vi "find_element(array).vi"(8 "error in (no error)":errorcluster, 10 "name":string, 11 "data store (in)":cluster{"name":string, "address":string}[](array[cluster])) -> (0 "error out":errorcluster, 1 "element":cluster{"name":string, "address":string}, 2 "element found ?":bool, 3 "data store (out)":cluster{"name":string, "address":string}[](array[cluster]))   [LabVIEW 2018]
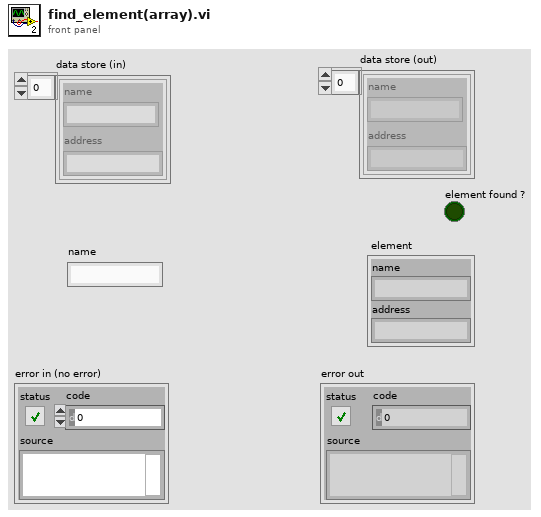
[diagram p1: front panel]
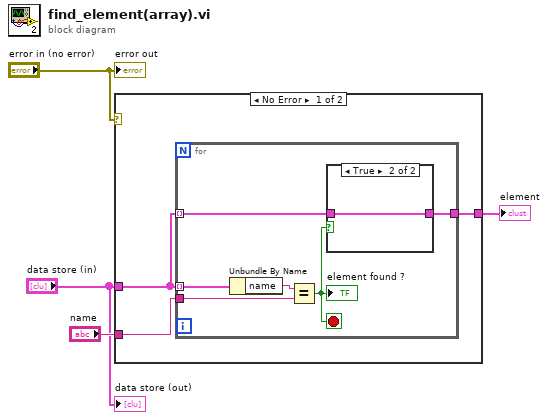
[diagram p0: block diagram]
diagram:
  n1 = case shown="No Error" "error in (no error)" {
    tunnel: "data store (in)" -> [w6 _]
    tunnel: "name" -> [w7 _]
    tunnel: [w5 _] -> w2
    frame No Error {
      n2 = for {
        tunnel: w6 -> [w13] mode=indexing
        tunnel: w7 -> [w11]
        tunnel: w6 -> [w10] mode=indexing
        tunnel: [w8] -> w5
        stop <- w9 stop-if-true
        n3 = Unbundle By Name(w13) -> ("name"=w12:string)
        n4 = Equal?(x=w12, y=w11) -> (x = y?=w9:bool)
        "element found ?" <- w9
        n5 = case shown="True" w9 {
          tunnel: w10 -> [_ w14]
          tunnel: [_ w14] -> w8
          frame False {
          }
          frame True {
          }
        }
      }
    }
    frame Error {
    }
  }
  "element" <- w2
  "error out" <- "error in (no error)"
  "data store (out)" <- "data store (in)"
